vi "Convert String to Hex.vi"(9 "bits per element":i32=4 min=1 max=64, 10 "Input String":string) -> (3 "Hex Values":u8[](array[numeric]) format="%.0x")   [LabVIEW 2011]
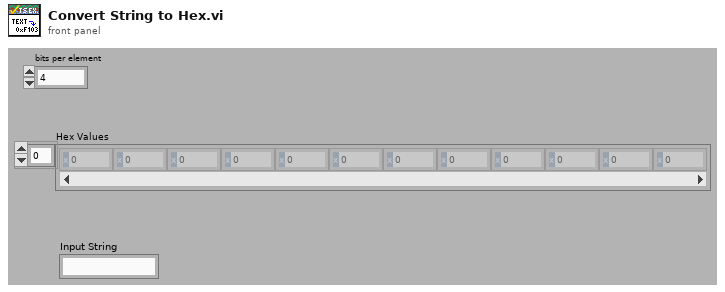
[diagram p1: front panel]
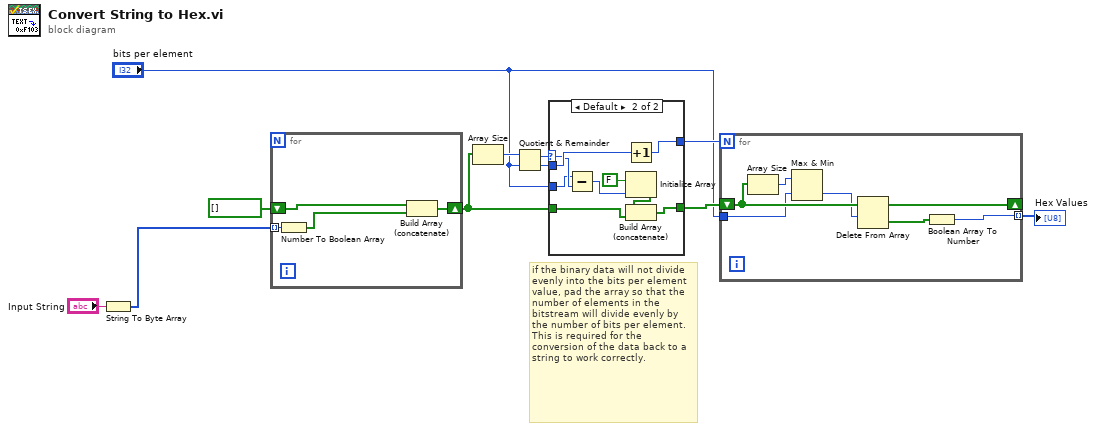
[diagram p0: block diagram]
diagram:
  # "if the binary data will not divide evenly into the bits per element value, pad the array so that the number of elements in the bitstream will divide evenly by the number of bits per element. This is required for the conversion of the data back to a string to work correctly."
  n1 = String To Byte Array(string="Input String") -> (unsigned byte array=w10:u8[])
  n2 = for {
    tunnel: w10 -> [w15] mode=indexing
    shift-right: [w14] -> w3
    shift-left: bool[] [] -> [w13]
    n3 = Number To Boolean Array(number=w15) -> (Boolean array=w12:bool[])
    n4 = Build Array (concatenate)(w13, w12) -> (w14:bool[])
  }
  n5 = Array Size(array=w3) -> (size(s)=w7:i32)
  n6 = Quotient & Remainder(x=w7, y="bits per element") -> (x-y*floor(x/y)=w6:i32, floor(x/y)=w5:i32)
  n7 = case shown="Default" w6 {
    selector: w6 -> [_ w20]
    tunnel: w5 -> [w17 w21]
    tunnel: [w17 w26] -> w4
    tunnel: w3 -> [w16 w24]
    tunnel: [w16 w23] -> w2
    tunnel: "bits per element" -> [_ w19]
    frame 0 {
    }
    frame Default {
      n8 = Subtract(x=w19, y=w20) -> (x-y=w18:i32)
      n9 = Increment(x=w21) -> (x+1=w26:i32)
      n10 = Initialize Array(FALSE, w18) -> (w22:bool[])
      n11 = Build Array (concatenate)(w22, w24) -> (w23:bool[])
    }
  }
  n12 = for {
    N: w4 -> [_]
    tunnel: "bits per element" -> [w29]
    shift-right: [w32] -> _
    shift-left: w2 -> [w31]
    tunnel: [w33] -> w8 mode=indexing
    n13 = Array Size(array=w31) -> (size(s)=w30:i32)
    n14 = Max & Min(x=w30, y=w29) -> (min(x,y)=w28:i32)  [unwired: 1 out]
    n15 = Delete From Array(array=w31, length=w28) -> (deleted portion=w27:bool[], array with subset deleted=w32:bool[])  [unwired: 1 in]
    n16 = Boolean Array To Number(Boolean array=w27) -> (number=w33:u32)
  }
  "Hex Values" <- w8
